vi "DeviceConnectionInfoUpdateRoutedMessage_Create.vi"(7 "Header":T2, 8 "error in (no error)":errorcluster, 10 "SendTo":string, 11 "DeviceConnectionInfoUpdateRoutedMessage":T1) -> (0 "error out":errorcluster, 3 "Message":T4)   [LabVIEW 2017]
uses:
  <vilib>/addons/InsightCM/MessageBus/Base/controls/Message.ctl
  <vilib>/addons/InsightCM/MessageBus/Base/controls/MessageHeader.ctl
  <vilib>/addons/InsightCM/MessageBus/Base/controls/KeyValuePair.ctl
  <vilib>/addons/InsightCM/MessageBus/MessageLibrary/Device/controls/DeviceConnectionInfoUpdateRoutedMessageBody.ctl
  <vilib>/addons/InsightCM/MessageBus/Base/controls/MessageClassType.ctl
  <vilib>/addons/InsightCM/Utilities/PropertyHelpers/PropertyHelpers.lvlib
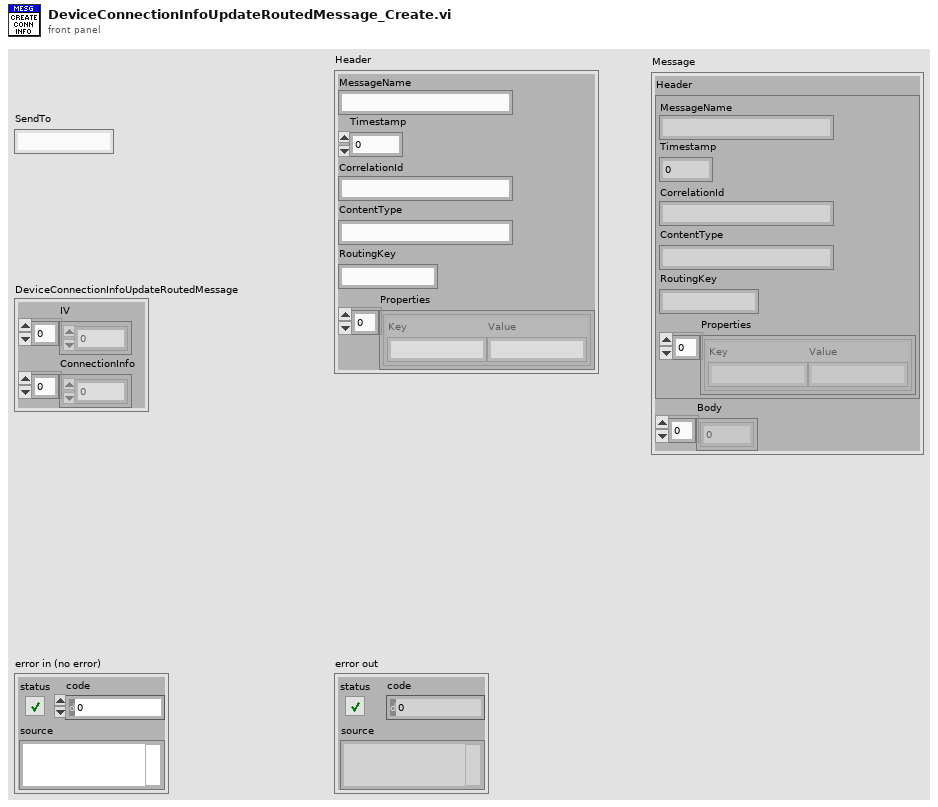
[diagram p1: front panel]
types:
  T1 = typedef "DeviceConnectionInfoUpdateRoutedMessageBody.ctl" = cluster{"IV":u8[], "ConnectionInfo":u8[]}
  T2 = typedef "MessageHeader.ctl" = cluster{"MessageName":string, "Timestamp":i64, "CorrelationId":string, "ContentType":string, "RoutingKey":string, "Properties":T3[]}
  T3 = typedef "KeyValuePair.ctl" = cluster{"Key":string, "Value":string}
  T4 = typedef "Message.ctl" = cluster{"Header":T2, "Body":u8[]}
  T5 = typedef "MessageClassType.ctl" = enum16{"Request", "Response", "Broadcast", "RoutedMessage"}
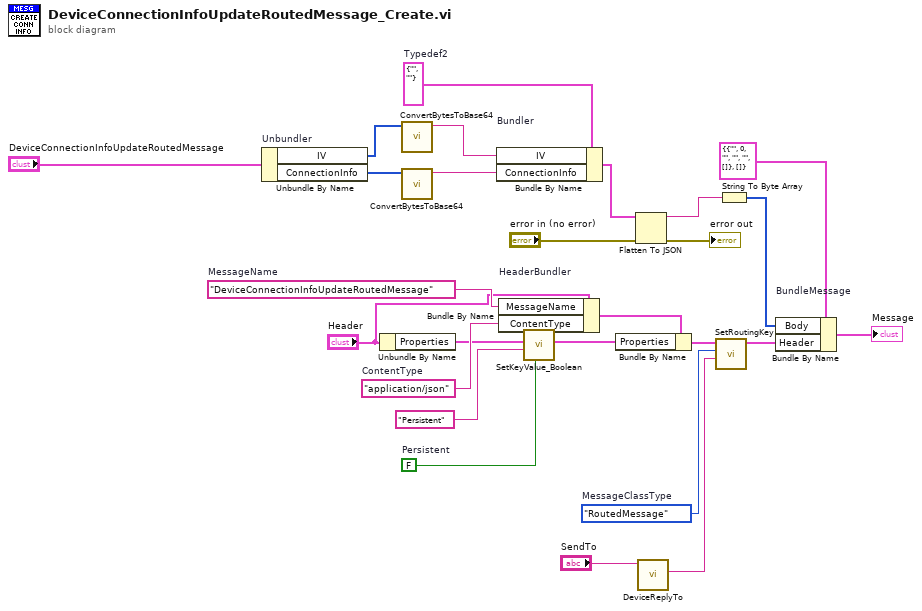
[diagram p0: block diagram]
diagram:
  w5 = cluster{"IV":string, "ConnectionInfo":string} {"IV"="", "ConnectionInfo"=""}  # Typedef2
  w22 = MessageClassType."RoutedMessage"  # MessageClassType
  w17 = FALSE  # Persistent
  w23 = "DeviceConnectionInfoUpdateRoutedMessage"  # MessageName
  w20 = "application/json"  # ContentType
  n1 = Unbundle By Name "Unbundler"("DeviceConnectionInfoUpdateRoutedMessage") -> ("IV"=w4:u8[], "ConnectionInfo"=w2:u8[])
  n2 = Unbundle By Name("Header") -> ("Properties"=w19:T3[])
  n3 = call <vilib>:"ConvertBytesToBase64.vi"("U8 array"=w4) -> ("base64 encoded"=w3:string)  [unwired: 10 in]
  n4 = call <vilib>:"ConvertBytesToBase64.vi"("U8 array"=w2) -> ("base64 encoded"=w1:string)  [unwired: 10 in]
  n5 = Bundle By Name "Bundler"(cluster=w5, "IV"=w3, "ConnectionInfo"=w1) -> (w6:cluster{"IV":string, "ConnectionInfo":string})
  n6 = Bundle By Name "HeaderBundler"(cluster="Header", "MessageName"=w23, "ContentType"=w20) -> (w14:T2)
  n7 = call <vilib>:"SetKeyValue_Boolean.vi"("value"=w17, "key"="Persistent" ("Key"), "key value pairs"=w19) -> ("key value pairs out"=w13:T3[])  [unwired: 8 in]
  n8 = Bundle By Name(cluster=w14, "Properties"=w13) -> (w15:T2)
  n9 = Flatten To JSON(anything=w6, error in (no error)="error in (no error)") -> (JSON string=w8:string, 11:→"error out":errorcluster)  [unwired: 1 in]
  n10 = call <vilib>:"DeviceReplyTo.vi"("Device"="SendTo") -> ("ReplyTo"=w9:string)  [unwired: 10 in]
  n11 = call <vilib>:"SetRoutingKey.vi"("SendTo"=w9, "MessageClassType"=w22, "Message Header in"=w15) -> ("Message Header out"=w16:T2)  [unwired: 8 in]
  n12 = String To Byte Array(string=w8) -> (unsigned byte array=w25:u8[])
  n13 = Bundle By Name "BundleMessage"(cluster=T4 {"Header"={"MessageName"="", "Timestamp"=0, "CorrelationId"="", "ContentType"="", "RoutingKey"="", "Properties"=[]}, "Body"=[]} ("Message"), "Body"=w25, "Header"=w16) -> (→"Message":T4)
